vi "MB_Read_Register_v2.vi"(0 "MB session in":refnum<class "MB_Master.lvclass">, 1 "starting address":u16=35116, 7 "ganho":dbl[](array[numeric]), 9 "error in (no error)":errorcluster, 12 "quantity":u16=1) -> (4 "Registers":u16[](array[numeric]), 5 "MB session out":refnum<class "MB_Master.lvclass">, 11 "error out":errorcluster)   [LabVIEW 2025]
uses:
  <vilib>/Plasmionique/MB Master/MB_Master/MB_Master.lvclass
  <vilib>/Plasmionique/MB Master/MB Master.lvlib
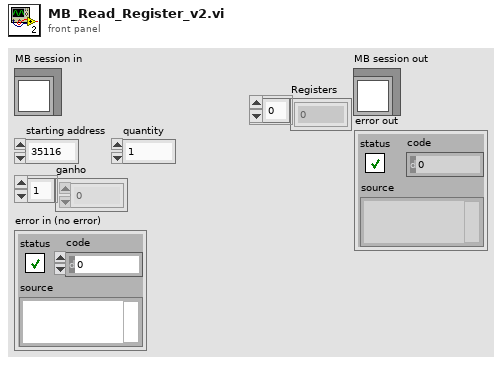
[diagram p1: front panel]
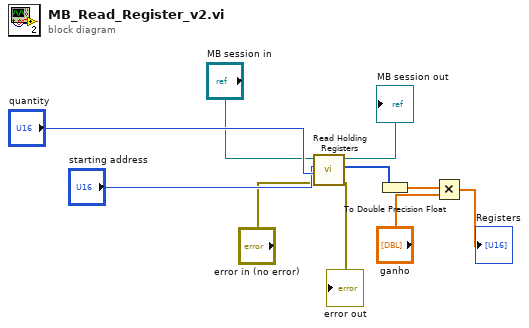
[diagram p0: block diagram]
diagram:
  n1 = call <vilib>:"Read Holding Registers.vi"("error in (no error)"="error in (no error)", "quantity"="quantity", "starting address"="starting address", "MB session in"="MB session in") -> ("error out"=→"error out":errorcluster, "Registers"=w6:u16[], "MB session out"=→"MB session out":refnum<class "MB_Master.lvclass">)  [unwired: 5 in]
  n2 = To Double Precision Float(number=w6) -> (double precision float=w5:dbl[])
  n3 = Multiply(x=w5, y="ganho") -> (x*y=→"Registers":dbl[])
